vi "Prepare queue for message (SubVI).vi"(5 "Connection in":refnum<class "Connection.lvclass">, 6 "error in (no error)":errorcluster, 7 "binding key":string[](array[string])=["broadcast.#"], 8 "exchange name":u16(ring) items=["requests", "alerts"], 9 "queue \nname":string) -> (0 "error out":errorcluster, 1 "Exchange.lvclass":refnum<class "Exchange.lvclass">, 2 "Queue out":refnum<class "Queue.lvclass">, 3 "Channel out":refnum<class "Channel.lvclass">, 4 "Connection out":refnum<class "Connection.lvclass">)   [LabVIEW 2016]
doc: "Create an exchange, a queue and add a list of bindings to this queue.\nThe properties of the queue follows dripline standard (auto-delete and eclusive)."
uses:
  <vilib>/Distrio/LabbitMQ/Connection/Connection.lvclass
  <vilib>/Distrio/LabbitMQ/Queue/Queue.lvclass
  <vilib>/Distrio/LabbitMQ/Exchange/Exchange.lvclass
  <vilib>/Distrio/LabbitMQ/Channel/Channel.lvclass
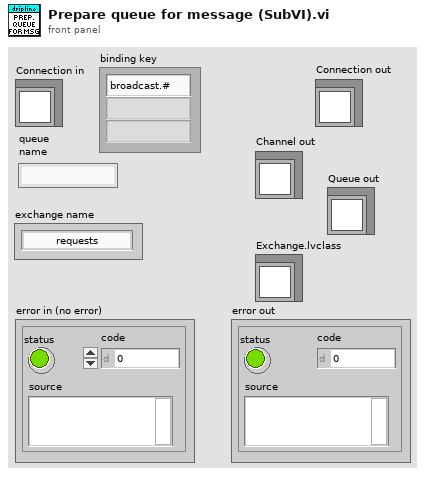
[diagram p1: front panel]
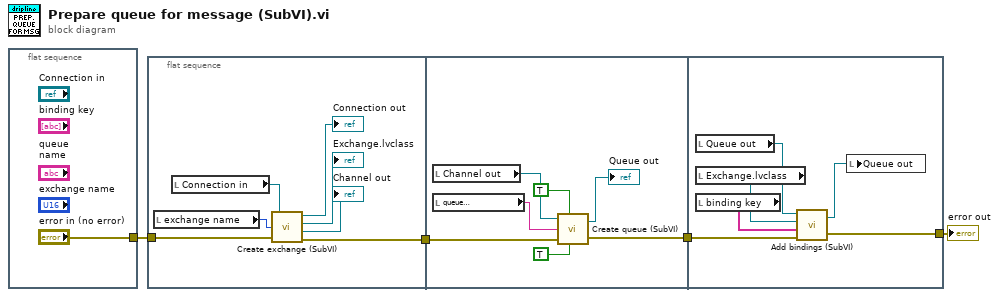
[diagram p0: block diagram]
diagram:
  n1 = flat-sequence {
    tunnel: ["error in (no error)"] -> w4
    frame #0 {
    }
  }
  n2 = flat-sequence {
    tunnel: w4 -> [w12]
    tunnel: [w11] -> w3
    tunnel: w3 -> [w19]
    tunnel: [w18] -> w2
    tunnel: w2 -> [w25]
    tunnel: [w24] -> w1
    frame #0 {
      n3 = local read "exchange name"() -> (w9:u16)
      n4 = local read "Connection in"() -> (w10:refnum<class "Connection.lvclass">)
      n5 = call "Create exchange (SubVI).vi"("Connection in"=w10, "exchange name"=w9, "error in (no error)"=w12) -> ("Connection out"=→"Connection out":refnum<class "Connection.lvclass">, "Exchange.lvclass"=→"Exchange.lvclass":refnum<class "Exchange.lvclass">, "Channel out"=→"Channel out":refnum<class "Channel.lvclass">, "error out"=w11:errorcluster)
    }
    frame #1 {
      n6 = local read "Channel out"() -> (w17:refnum<class "Channel.lvclass">)
      n7 = local read "queue \nname"() -> (w16:string)
      n8 = call "Create queue (SubVI).vi"("Channel in"=w17, "autoDelete (F)"=TRUE, "queue"=w16, "error in (no error)"=w19, "exclusive (F)"=TRUE) -> ("Queue out"=→"Queue out":refnum<class "Queue.lvclass">, "error out"=w18:errorcluster)
    }
    frame #2 {
      n9 = local read "Queue out"() -> (w23:refnum<class "Queue.lvclass">)
      n10 = local read "Exchange.lvclass"() -> (w22:refnum<class "Exchange.lvclass">)
      n11 = local read "binding key"() -> (w21:string[])
      n12 = call "Add bindings (SubVI).vi"("error in (no error)"=w25, "binding key"=w21, "Exchange.lvclass"=w22, "Queue in"=w23) -> ("error out"=w24:errorcluster, "Queue out"=w20:refnum<class "Queue.lvclass">)
      n13 = local write "Queue out"(w20) -> ()
    }
  }
  "error out" <- w1
